vi "Cell gas meter display.vi"() -> ()   [LabVIEW 2015]
uses:
  Libraries/HeliumMonitor/Sensor configuration.ctl
  Libraries/HeliumMonitor/Channel type.ctl
  <vilib>/Platform/TimedLoop/XDataNode/timing_clust.ctl
  <vilib>/Platform/TimedLoop/XDataNode/nitl_modes.ctl
  <vilib>/Platform/TimedLoop/XDataNode/wakeup.ctl
  <vilib>/platform/TimedLoop/XDataNode/XDataNode.xnode
  <vilib>/Platform/TimedLoop/XDataNode/XDNodeRunTimeDep.lvlib
panel:
  in  "Tab Control":enum32{"Plot", "Configuration"}(tab)
  in  "Gas/Liquid?":bool
  out "Cell 4":cluster{dbl[], dbl[]}[](graph) caption="Optics lab"
  out "Total  Liters":dbl
  out "Trip  Liters":dbl
  in  "Reset trip":bool
  out "Trip rest time":timestamp format="%<%H:%M:%S\n%x>T"
  out "Trip  Liters 2":dbl caption="Trip Liquid (Liters)" format="%#.1f"
  out "Total  Liters 2":dbl caption="Total Liquid (Liters)" format="%#.1f"
  in  "Sensor configuration":T1={"Name"="Optics lab", "URL"="http:\\\\130.55.69.44", "Channels"=[{"type"=enum."Flow meter", "number"=6.0}]}
  out "Subtract liters":i32
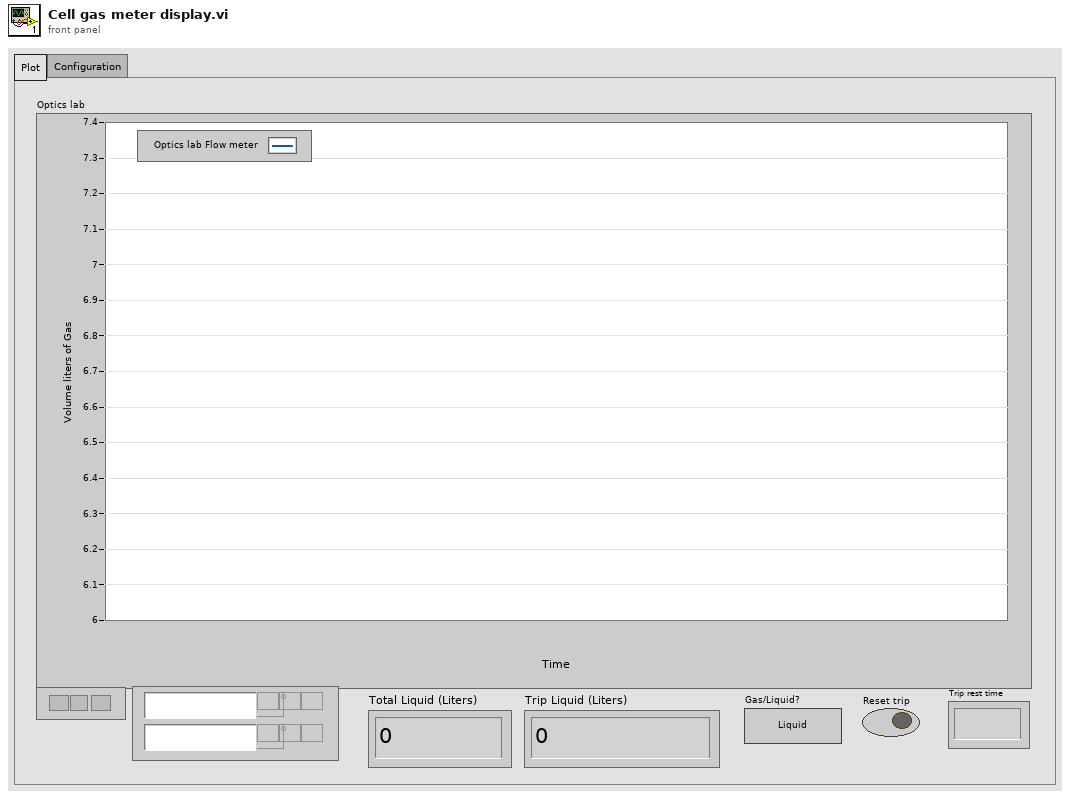
[diagram p1: front panel]
types:
  T1 = typedef "Sensor configuration.ctl" = cluster{"Name":string, "URL":string, "Channels":cluster{"type":T2, "number":dbl}[]}
  T2 = typedef "Channel type.ctl" = enum16{"Volts", "Flow meter", "Tank pressure", "Dewar level", "Raw ADC"}
  T3 = typedef "XDNodeRunTimeDep.lvlib/timing_clust.ctl" = cluster{"Expected End [f-1]":u64, "Actual End [f-1]":u64, "Finished Late? [f-1]":bool, "Expected End [i-1]":u64, "Actual End [i-1]":u64, "Finished Late? [i-1]":bool, "Expected Start [i]":u64, "Actual Start [i]":u64, "Expected Start [f]":u64, "Actual Start [f]":u64, "Source Name":string, "Structure Name":string, "Period":i64, "Deadline":i64, "Offset":i64, "Start":i64, "Priority":i32, "Timeout":i32, "Mode":T4, "Wakeup Reason":T5, "Error":errorcluster, "Source Type":string, "Secondary Source Type":string, "Global End Time":u64, "Global Start Time":u64, "Frame Duration":u64, "Iteration Duration":u64, "Assigned CPU":i32, "I/O Scan Engine Mode":u32}
  T4 = typedef "XDNodeRunTimeDep.lvlib/nitl_modes.ctl" = enum32{"No Change", "Process missed periods, maintain original phase", "Discard missed periods, maintain original phase", "Process missed periods, ignore original phase", "Discard missed periods, ignore original phase"}
  T5 = typedef "XDNodeRunTimeDep.lvlib/wakeup.ctl" = enum32{"Normal", "Aborted", "Asynchronous wakeup", "Timing source error", "Timed loop error", "Timeout"}
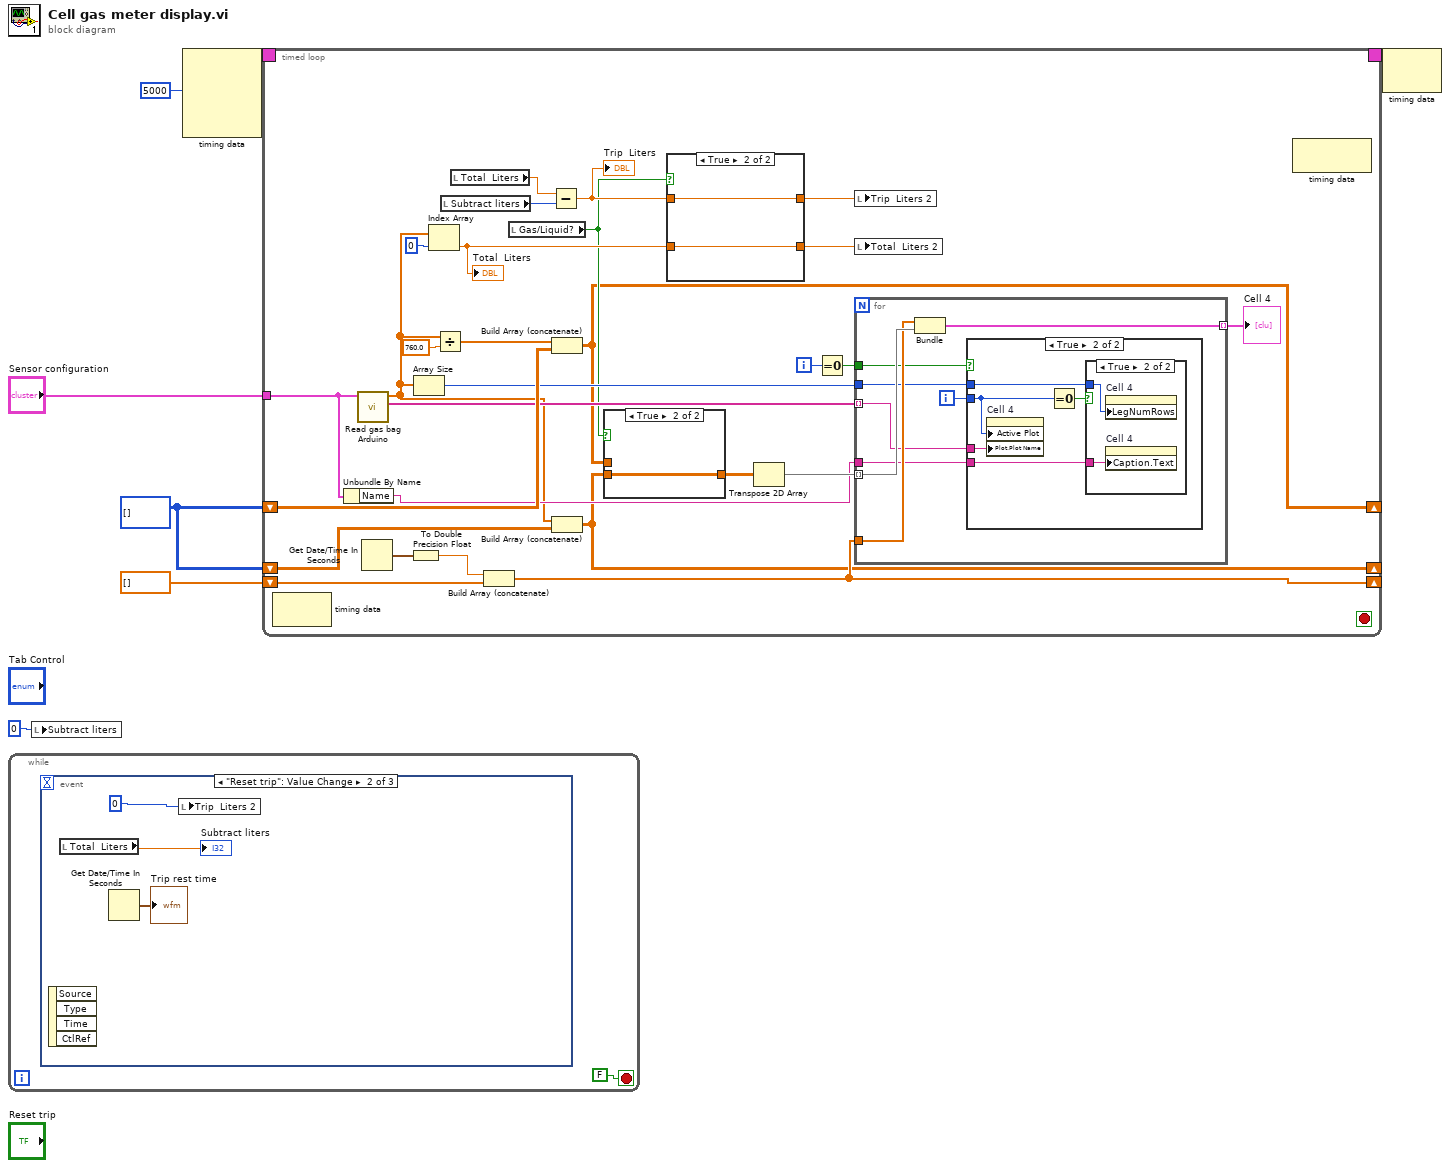
[diagram p0: block diagram]
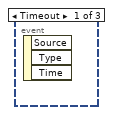
[diagram p2: hidden frame]
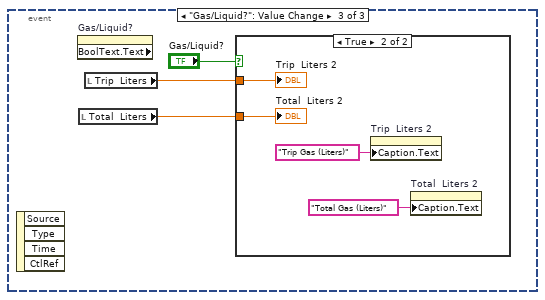
[diagram p3: hidden frame]
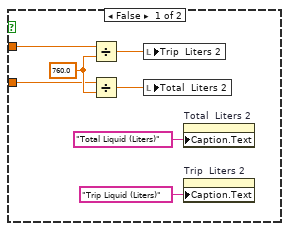
[diagram p4: hidden frame]
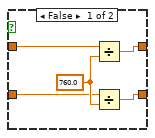
[diagram p6: hidden frame]
diagram:
  w1 = i32[][] []
  n1 = while {
    stop <- FALSE stop-if-true
    n2 = event shown="[1] \"Reset trip\": Value Change" {
      selector: _ -> [_ _ _]
      dyn-events: _ -> [_ _ _]
      timeout: _ -> [_ _ _]
      event Timeout {
        n3 = event-data() -> ()  [unwired: 1 in, 3 out]
      }
      event "Reset trip": Value Change {
        n4 = event-data() -> ()  [unwired: 1 in, 4 out]
        n5 = local read "Total  Liters"() -> (→"Subtract liters":dbl)
        n6 = Get Date/Time In Seconds() -> (seconds since 1Jan1904=→"Trip rest time":timestamp)
        n7 = local write "Trip  Liters 2"(0 ("Trip Liters")) -> ()
      }
      event "Gas/Liquid?": Value Change {
        n8 = event-data() -> ()  [unwired: 1 in, 4 out]
        n9 = property on="Gas/Liquid?" class="Bool (strict)" props=["BoolText", "Text"]() -> ()  [unwired: 2 in, 3 out]
        n10 = local read "Total  Liters"() -> (w12:dbl)
        n11 = local read "Trip  Liters"() -> (w13:dbl)
        n12 = case shown="True" "Gas/Liquid?" {
          tunnel: w13 -> [w16 w23]
          tunnel: w12 -> [w15 w22]
          frame False {
            w19 = 760.0 ("y")
            n13 = Divide(x=w16, y=w19) -> (x/y=w20:dbl)
            n14 = Divide(x=w15, y=w19) -> (x/y=w21:dbl)
            n15 = local write "Trip  Liters 2"(w20) -> ()
            n16 = local write "Total  Liters 2"(w21) -> ()
            n17 = property on="Total  Liters 2" class="DigNum (strict)"("Caption.Text"="Total Liquid (Liters)") -> ()  [unwired: 2 in, 2 out]
            n18 = property on="Trip  Liters 2" class="DigNum (strict)"("Caption.Text"="Trip Liquid (Liters)") -> ()  [unwired: 2 in, 2 out]
          }
          frame True {
            n19 = property on="Trip  Liters 2" class="DigNum (strict)"("Caption.Text"="Trip Gas (Liters)") -> ()  [unwired: 2 in, 2 out]
            n20 = property on="Total  Liters 2" class="DigNum (strict)"("Caption.Text"="Total Gas (Liters)") -> ()  [unwired: 2 in, 2 out]
            "Trip  Liters 2" <- w23
            "Total  Liters 2" <- w22
          }
        }
      }
    }
  }
  n21 = local write "Subtract liters"(0 ("Subtract liters")) -> ()
  n22 = node-c288(i64 5000 ("Period")) -> (w7:T3)  [unwired: 3 in]
  n23 = timed-loop {
    timing: w7 -> [_]
    timing-out: [_] -> w6
    shift-right: [w46] -> _
    shift-left: dbl[] [] -> [w51]
    shift-right: [w26] -> _
    shift-left: w1 -> [w50]
    tunnel: "Sensor configuration" -> [w39]
    shift-right: [w29] -> _
    shift-left: w1 -> [w30]
    i -> [w40]
    stop <- _ stop-if-true
    n24 = node-c288() -> ()  [unwired: 1 in, 1 out]
    n25 = Unbundle By Name(w39) -> ("Name"=w38:string)
    n26 = call "Read gas bag Arduino.vi"("Sensor configuration"=w39) -> ("Data"=w31:dbl[], "Names"=w42:string[])  [unwired: 6 in, 2 out]
    n27 = Get Date/Time In Seconds() -> (seconds since 1Jan1904=w53:timestamp)
    n28 = To Double Precision Float(number=w53) -> (double precision float=w52:dbl)
    n29 = Array Size(array=w31) -> (size(s)=w43:i32)
    n30 = Index Array(array=w31, index=0 ("index (row)")) -> (element=w33:dbl)
    "Total  Liters" <- w33
    n31 = Divide(x=w31, y=760.0) -> (x/y=w37:dbl[])
    n32 = local read "Subtract liters"() -> (w47:i32)
    n33 = local read "Total  Liters"() -> (w48:dbl)
    n34 = Build Array (concatenate)(w52, w51) -> (w46:dbl[])
    n35 = local read "Gas/Liquid?"() -> (w27:bool)
    n36 = Subtract(x=w48, y=w47) -> (x-y=w32:dbl)
    "Trip  Liters" <- w32
    n37 = Build Array (concatenate)(w37, w50) -> (w26:dbl[][])
    n38 = Build Array (concatenate)(w31, w30) -> (w29:dbl[][])
    n39 = case shown="True" w27 {
      tunnel: w29 -> [_ w55]
      tunnel: [w54 w55] -> w28
      tunnel: w26 -> [w54 _]
      frame False {
      }
      frame True {
      }
    }
    n40 = case shown="True" w27 {
      tunnel: w32 -> [w59 w62]
      tunnel: w33 -> [w58 w61]
      tunnel: [w57 w62] -> w35
      tunnel: [w56 w61] -> w34
      frame False {
        w60 = 760.0 ("y")
        n41 = Divide(x=w59, y=w60) -> (x/y=w57:dbl)
        n42 = Divide(x=w58, y=w60) -> (x/y=w56:dbl)
      }
      frame True {
      }
    }
    n43 = Transpose 2D Array(2D array=w28) -> (transposed array=w44:dbl[][])
    n44 = Equal To 0?(x=w40) -> (x = 0?=w41:bool)
    n45 = local write "Trip  Liters 2"(w35) -> ()
    n46 = local write "Total  Liters 2"(w34) -> ()
    n47 = for {
      tunnel: w44 -> [w70] mode=indexing
      tunnel: w46 -> [w69]
      tunnel: [w68] -> w45 mode=indexing
      tunnel: w43 -> [w67]
      tunnel: w42 -> [w66] mode=indexing
      tunnel: w41 -> [w65]
      tunnel: w38 -> [w63]
      i -> [w64]
      n48 = Bundle(w69, w70) -> (w68:cluster{dbl[], dbl[]})  [unwired: 1 in]
      n49 = case shown="True" w65 {
        tunnel: w67 -> [_ w75]
        tunnel: w66 -> [_ w74]
        tunnel: w64 -> [_ w72]
        tunnel: w63 -> [_ w73]
        frame False {
        }
        frame True {
          n50 = property on="Cell 4" class="XYGraph (strict)"("Active Plot"=w72, "Plot.Plot Name"=w74) -> ()  [unwired: 2 in, 2 out]
          n51 = Equal To 0?(x=w72) -> (x = 0?=w71:bool)
          n52 = case shown="True" w71 {
            tunnel: w75 -> [_ w77]
            tunnel: w73 -> [_ w76]
            frame False {
            }
            frame True {
              n53 = property on="Cell 4" class="XYGraph (strict)"("LegNumRows"=w77) -> ()  [unwired: 2 in, 2 out]
              n54 = property on="Cell 4" class="XYGraph (strict)"("Caption.Text"=w76) -> ()  [unwired: 2 in, 2 out]
            }
          }
        }
      }
    }
    "Cell 4" <- w45
    n55 = node-c288() -> ()  [unwired: 1 in, 1 out]
  }
  n56 = node-c288(w6) -> ()  [unwired: 1 out]
